vi "MQTT_SSL_Connect.vi"(5 "Connect Meta":T7={"QoS"=enum."At most once", "DUP"=FALSE, "Retain"=TRUE, "Keep Alive (sec)"=60}, 6 "Client ID":string="LabVIEW_MQTT_Client", 7 "Connect Flags":T3, 8 "error in (no error)":errorcluster, 9 "Will Info":T8={"Will message"="Last Will", "Will Topic"="Will Topic"}, 10 "User Info":T9={"User Name"="User", "Password"="password"}, 11 "MQTT Broker":cluster{"address (IP)":string, "port":u16}={"address (IP)"="broker.mqttdashboard.com", "port"=1883}) -> (0 "error out":errorcluster, 2 "Connection Status":T10=enum."Connection refused: not authorized", 3 "SSL_Connection 2":T1)   [LabVIEW 2015, in "AWS_IoT.lvlib"]
uses:
  AWS_IoT.lvlib
  LVMQTT/Controls/Connection_Return_Codes.ctl
  LVMQTT/Controls/User_Info.ctl
  LVMQTT/Controls/Will_Info.ctl
  LVMQTT/Controls/QoS.ctl
  LVMQTT/Controls/DUP_Flag.ctl
  LVMQTT/Controls/Retain_Flag.ctl
  LVMQTT/Controls/Connect_Flags.ctl
  Controls/SSL_login.ctl
  Controls/SSL_Connection.ctl
  LVMQTT/Controls/MessageType.ctl
  LVMQTT/Controls/Conn_Stat_FGV_Cmds.ctl
  LVMQTT/MQTT_Functions.lvlib
panel:
  in  "SSL_Connection":T1
  in  "login":T2={"server IP"="", "server port"=0, "local port (0 = auto)"=0, "timeout ms (1000)"=1000}
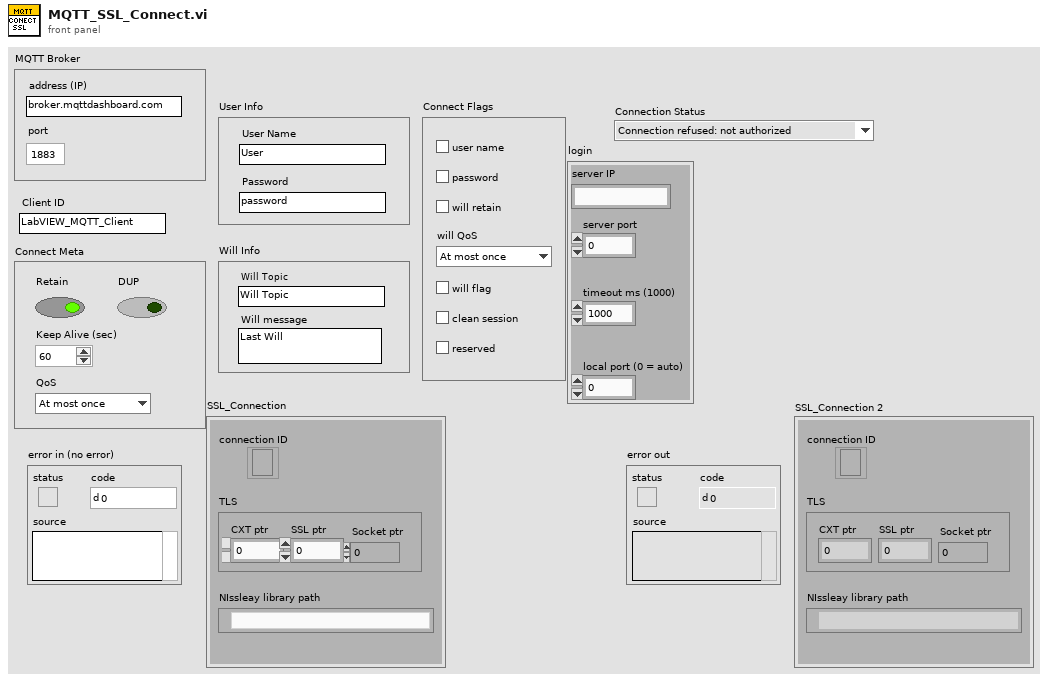
[diagram p1: front panel]
types:
  T1 = typedef "AWS_IoT.lvlib/SSL_Connection.ctl" = cluster{"connection ID":refnum<k5>, "TLS":cluster{"CXT ptr":i32, "SSL ptr":i32, "Socket ptr":u64}, "NIssleay library path":path}
  T2 = typedef "AWS_IoT.lvlib/SSL_login.ctl" = cluster{"server IP":string, "server port":u16, "local port (0 = auto)":u16, "timeout ms (1000)":i32}
  T3 = typedef "MQTT_Functions.lvlib/Connect_Flags.ctl" = cluster{"user name":bool, "password":bool, "will retain":bool, "will flag":bool, "clean session":bool, "reserved":bool, "will QoS":T4}
  T4 = typedef "MQTT_Functions.lvlib/QoS.ctl" = enum8{"At most once", "At least once", "Exactly once", "Reserved"}
  T5 = typedef "MQTT_Functions.lvlib/DUP_Flag.ctl" = bool
  T6 = typedef "MQTT_Functions.lvlib/Retain_Flag.ctl" = bool
  T7 = cluster{"QoS":T4, "DUP":T5, "Retain":T6, "Keep Alive (sec)":u16}
  T8 = typedef "MQTT_Functions.lvlib/Will_Info.ctl" = cluster{"Will message":string, "Will Topic":string}
  T9 = typedef "MQTT_Functions.lvlib/User_Info.ctl" = cluster{"User Name":string, "Password":string}
  T10 = typedef "MQTT_Functions.lvlib/Connection_Return_Codes.ctl" = enum16{"Connection accepted", "Connection refused: unacceptable protocol version", "Connection refused: identifier rejected", "Connection refused: Server unavailable", "Connection refused: bad user name or password", "Connection refused: not authorized"}
  T11 = typedef "MQTT_Functions.lvlib/Conn_Stat_FGV_Cmds.ctl" = enum16{"Get", "Set"}
  T12 = typedef "MQTT_Functions.lvlib/MessageType.ctl" = enum32{"Reserved", "CONNECT", "CONNACK", "PUBLISH", "PUBACK", "PUBREC", "PUBREL", "PUBCOMP", "SUBSCRIBE", "SUBACK", "UNSUBSCRIBE", "UNSUBACK", "PINGREQ", "PINGRESP", "DISCONNECT", "Reserved2"}
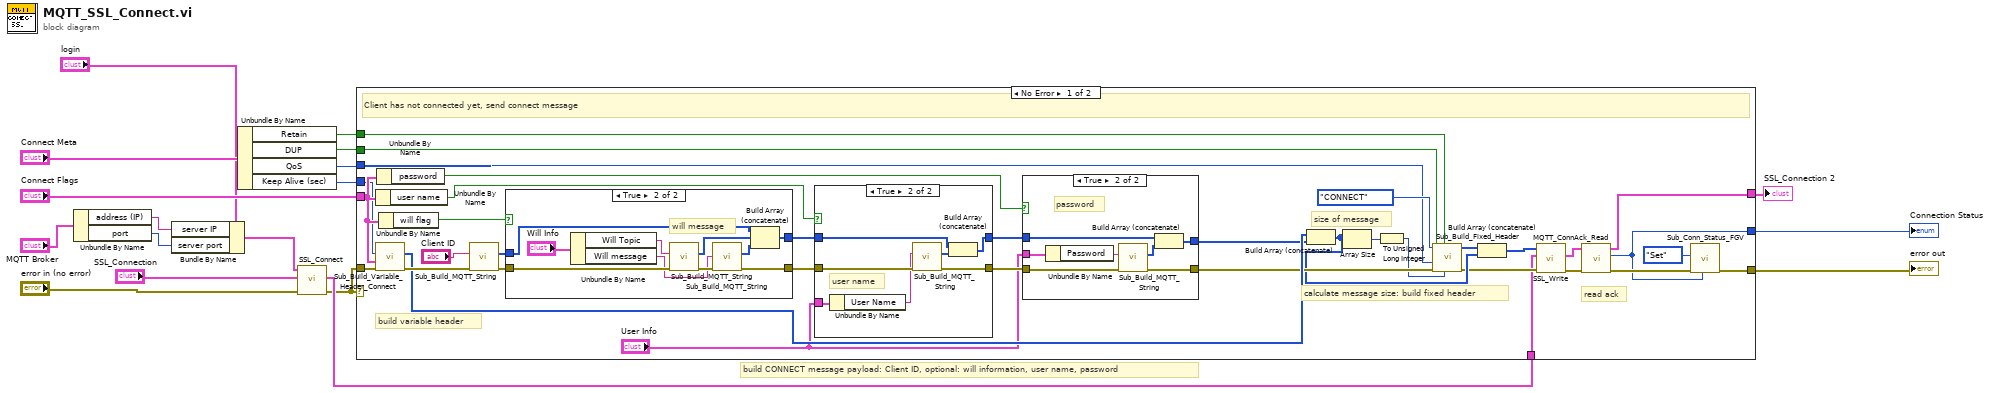
[diagram p0: block diagram]
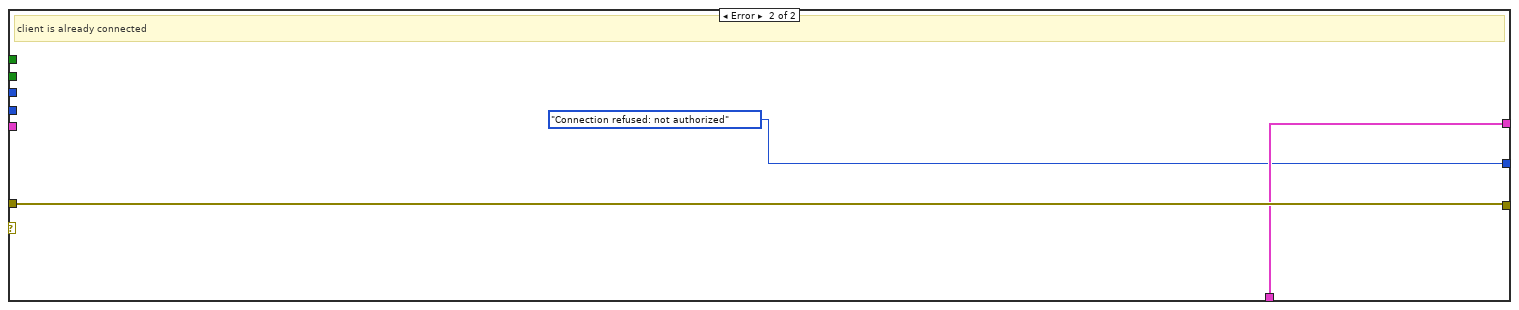
[diagram p5: hidden frame]
diagram:
  # "build CONNECT message payload: Client ID, optional: will information, user name, password"
  n1 = Unbundle By Name("MQTT Broker") -> ("address (IP)"=w6:string, "port"=w5:u16)
  n2 = Bundle By Name(cluster="login", "server IP"=w6, "server port"=w5) -> (w9:T2)
  n3 = Unbundle By Name("Connect Meta") -> ("Retain"=w13:T6, "DUP"=w14:T5, "QoS"=w15:T4, "Keep Alive (sec)"=w16:u16)
  n4 = call "SSL_Connect.vi"("error in (no error)"="error in (no error)", "SSL_Connection"="SSL_Connection", "login"=w9) -> ("error out"=w1:errorcluster, "SSL_Connection"=w3:T1)  [unwired: 7 in]
  n5 = case shown="No Error" w1 {
    tunnel: "Connect Flags" -> [w48 _]
    tunnel: w13 -> [w34 _]
    tunnel: w14 -> [w33 _]
    tunnel: w15 -> [w32 _]
    tunnel: w16 -> [w31 _]
    tunnel: w1 -> [w26 w87]
    tunnel: w3 -> [w20 w86]
    tunnel: [w22 w87] -> w17
    tunnel: [w21 Connection_Return_Codes."Connection refused: not authorized" ("Connection Status")] -> w18
    tunnel: [w25 w86] -> w2
    frame No Error {
      # "read ack"
      # "calculate message size: build fixed header"
      # "build variable header"
      # "size of message"
      # "Client has not connected yet, send connect message"
      n6 = Unbundle By Name(w48) -> ("user name"=w47:bool)
      n7 = call "Sub_Build_Variable_Header_Connect.vi"("error in (no error)"=w26, "Connect Flags"=w48, "Keep Alive (sec)"=w31) -> ("error out"=w53:errorcluster, "Variable Header"=w44:u8[])  [unwired: 7 in]
      n8 = Unbundle By Name(w48) -> ("password"=w46:bool)
      n9 = Unbundle By Name(w48) -> ("will flag"=w45:bool)
      n10 = call "Sub_Build_MQTT_String.vi"("error in (no error)"=w53, "String to be encoded"="Client ID") -> ("error out"=w49:errorcluster, "UTF8 Byte Array"=w52:u8[])  [unwired: 8 in]
      n11 = case shown="True" w45 {
        tunnel: w52 -> [w74 w82]
        tunnel: [w74 w83] -> w51
        tunnel: w49 -> [w73 w81]
        tunnel: [w73 w78] -> w42
        frame False {
        }
        frame True {
          # "will message"
          n12 = Unbundle By Name("Will Info") -> ("Will Topic"=w76:string, "Will message"=w75:string)
          n13 = call "Sub_Build_MQTT_String.vi"("error in (no error)"=w81, "String to be encoded"=w76) -> ("error out"=w80:errorcluster, "UTF8 Byte Array"=w79:u8[])  [unwired: 8 in]
          n14 = call "Sub_Build_MQTT_String.vi"("error in (no error)"=w80, "String to be encoded"=w75) -> ("error out"=w78:errorcluster, "UTF8 Byte Array"=w84:u8[])  [unwired: 8 in]
          n15 = Build Array (concatenate)(w82, w79, w84) -> (w83:u8[])
        }
      }
      n16 = case shown="True" w47 {
        tunnel: w51 -> [w65 w71]
        tunnel: [w65 w70] -> w50
        tunnel: [w64 w69] -> w43
        tunnel: w42 -> [w64 w68]
        tunnel: "User Info" -> [_ w67]
        frame False {
        }
        frame True {
          # "user name"
          n17 = Unbundle By Name(w67) -> ("User Name"=w66:string)
          n18 = call "Sub_Build_MQTT_String.vi"("error in (no error)"=w68, "String to be encoded"=w66) -> ("error out"=w69:errorcluster, "UTF8 Byte Array"=w72:u8[])  [unwired: 8 in]
          n19 = Build Array (concatenate)(w71, w72) -> (w70:u8[])
        }
      }
      n20 = case shown="True" w46 {
        tunnel: w50 -> [w56 w62]
        tunnel: [w56 w61] -> w40
        tunnel: w43 -> [w55 w60]
        tunnel: [w55 w59] -> w41
        tunnel: "User Info" -> [_ w58]
        frame False {
        }
        frame True {
          # "password"
          n21 = Unbundle By Name(w58) -> ("Password"=w57:string)
          n22 = call "Sub_Build_MQTT_String.vi"("error in (no error)"=w60, "String to be encoded"=w57) -> ("error out"=w59:errorcluster, "UTF8 Byte Array"=w63:u8[])  [unwired: 8 in]
          n23 = Build Array (concatenate)(w62, w63) -> (w61:u8[])
        }
      }
      n24 = Build Array (concatenate)(w44, w40) -> (w39:u8[])
      n25 = Array Size(array=w39) -> (size(s)=w37:i32)
      n26 = To Unsigned Long Integer(number=w37) -> (unsigned 32bit integer=w36:u32)
      n27 = call "Sub_Build_Fixed_Header.vi"("Remaining Length"=w36, "Retain"=w34, "error in (no error)"=w41, "QoS"=w32, "DUP"=w33, "MessageType"=MessageType."CONNECT") -> ("error out"=w29:errorcluster, "Fixed Header"=w38:u8[])  [unwired: 4 in]
      n28 = Build Array (concatenate)(w38, w39) -> (w28:u8[])
      n29 = call "SSL_Write.vi"("error in (no error)"=w29, "SSL_Connection"=w20, "data in"=w28) -> ("error out"=w27:errorcluster, "SSL_Connection"=w19:T1)  [unwired: 7 in]
      n30 = call "MQTT_ConnAck_Read.vi"("error in (no error)"=w27, "SSL_Connection"=w19) -> ("error out"=w24:errorcluster, "Connection Status"=w21:T10, "SSL_Connection 2"=w25:T1)  [unwired: 5 in, 2 out]
      n31 = call "Sub_Conn_Status_FGV.vi"("Connection Status in"=w21, "error in"=w24, "Command"=Conn_Stat_FGV_Cmds."Set") -> ("error out"=w22:errorcluster)  [unwired: 7 in, 1 out]
    }
    frame Error {
      # "client is already connected"
    }
  }
  "error out" <- w17
  "Connection Status" <- w18
  "SSL_Connection 2" <- w2
